vi "PH_Sixpack.Action Reset.vi"(0 "i ref in":refnum<vi>, 5 "error in":errorcluster) -> (14 "i ref out":refnum<vi>, 19 "error out":errorcluster)   [LabVIEW 2014, in "PH_Sixpack.lvlib"]
doc: "This VI resets the 6P."
uses:
  PH_Sixpack.lvlib
  PH_Sixpack.Status.ctl
  instr.lib/SixPack/Sixpack - Driver.lvlib
  PH_Stepmotor_BaseClass/PH_Stepmotor_BaseClass.lvlib
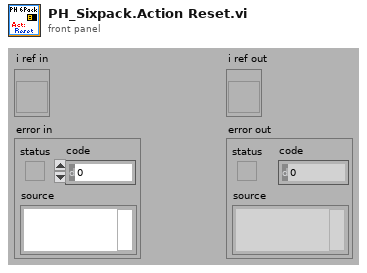
[diagram p1: front panel]
types:
  T1 = typedef "PH_Sixpack.lvlib/PH_Sixpack.Status.ctl" = enum32{"None", "Init", "Configure", "configured", "Close", "closed"}
  T2 = typedef "PH_Stepmotor_BaseClass.lvlib/PH_Stepmotor_BaseClass.i attribute.ctl" = cluster{"Device Error":errorcluster, "Axes PSDB Thread":cluster{"Ref":refnum<vi>, "Q-Ref":refnum<queue>, "Data Status":T3}, "Axes":T4[], "Axes PSDB Infos":cluster{"GUI Name":string, "PSDB Instance ID":i32, "PSDB Status Service ID":i32, "Axis":i32, "Class":string}[], "GUI Refs":T9}
  T3 = typedef "PH_PSDBWriter.lvlib/PH_PSDBWriter.Data Status.ctl" = i16
  T4 = typedef "PH_Stepmotor_BaseClass.lvlib/PH_Stepmotor_BaseClass.Axis Attributes.ctl" = cluster{"Settings":T5, "Endswitch?":bool, "DIM Service IDs":T7, "Activity":T8, "Configured?":bool, "Position":cluster{"Current":i32, "Target":i32}, "Position to set":cluster{"New?":bool, "Wanted":i32}, "Stop?":bool, "Reset?":bool, "Move?":bool, "Nothing connected?":bool}
  T5 = typedef "PH_Stepmotor_BaseClass.lvlib/PH_Stepmotor_BaseClass.Axis Settings.ctl" = cluster{"Sign change":bool, "Width":dbl, "Calibration":dbl, "Unit":string, "Motor Type":T6, "Unit Width":string, "Unit CF":string}
  T6 = typedef "PH_Stepmotor_BaseClass.lvlib/PH_Stepmotor_BaseClass.Motor Type.ctl" = enum16{"Unspecific", "OWIS 49.120.2633", "OWIS 49.060.1033", "OWIS 43.040.2558", "Diamond Motion 2200 series", "OWIS 49.120.266B.MV6", "Calorimeter", "Linear Stage 1", "MICOS VT-80", "MICOS VT-80 S", "Standa Rotstage nt0.95A", "PUF RA 320.200", "PUF RA 800.200", "PUF RA 800.400", "PUF RA 400.50", "1324.nn.800.50", "1324.n9c.800.50", "1324.nn.320.200", "1324.nn.400.200", "1324.nn.800.200", "1324.nn.400.50", "1324.8c9c.800.50", "1324.8c9c.400.200"}
  T7 = typedef "PH_Stepmotor_BaseClass.lvlib/PH_Stepmotor_BaseClass.Axis DIM Service IDs.ctl" = cluster{"Settings":i32, "Information":i32}
  T8 = typedef "PH_Stepmotor_BaseClass.lvlib/PH_Stepmotor_BaseClass.Axis Activity.ctl" = enum16{"No Information", "stopped", "running", "Failure", "Alarm", "stopped at backward ES", "stopped at foreward ES"}
  T9 = typedef "PH_Stepmotor_BaseClass.lvlib/PH_Stepmotor_BaseClass.GUI Refs.ctl" = cluster{"Axes Configuration":refnum<vi>, "Device Error":refnum<vi>, "Axes PSDB Infos":refnum<vi>}
  T10 = typedef "PH_Sixpack.lvlib/PH_Sixpack.i attribute.ctl" = cluster{"Information":cluster{"SixPack ID(0)":u16, "BaudRate(19200)":u16, "COM Port":enum32{"COM1", "COM2", "COM3", "COM4", "COM5", "COM6", "COM7", "COM8", "COM9"}, "HANDLE":i32}, "Serial Number":dbl, "Firmwareversion":dbl, "Axes":T11[], "Status":T1, "Axis to do a RefSearch":i32, "GUI Refs":cluster{"Information":refnum<vi>, "Serial Number":refnum<vi>, "Firmwareversion":refnum<vi>, "Status":refnum<vi>, "Axis to do a RefSearch":refnum<vi>, "Axes Configuration (Sixpack)":refnum<vi>, "Inputs":refnum<vi>, "PeriodicInterval [ms]":refnum<vi>}, "Constructor finished":bool, "Ignore Error":bool}
  T11 = typedef "PH_Sixpack.lvlib/PH_Sixpack.Axis Cluster.ctl" = cluster{"Config":T12, "To set?":cluster{"VmaxAmax":bool, "I max":bool, "VStartVminDivi":bool, "Ref Search Parameter":bool, "Stopswitch Limits":bool, "Axis Parameter":bool, "I Control":bool}}
  T12 = typedef "PH_Sixpack.lvlib/PH_Sixpack.Axis Configuration.ctl" = cluster{"VmaxAmax":T13, "I max (50%)":T14, "VStartVminDivi":T15, "Ref Search Parameter":T16, "Stopswitch Limits":T17, "Axis Parameter":T18, "I Control":T21}
  T13 = typedef "Sixpack - Driver.lvlib/VmaxAmax.ctl" = cluster{"VMax(511)":u16, "AMax(128)":u16}
  T14 = typedef "Sixpack - Driver.lvlib/PeakCurrent.ctl" = dbl
  T15 = typedef "Sixpack - Driver.lvlib/VStartVmin.ctl" = cluster{"VStart(5)":u16, "Vmin(4)":u16, "Div i (2)":enum8{"0", "1", "2", "3"}}
  T16 = typedef "Sixpack - Driver.lvlib/Ref Search Parameter.ctl" = cluster{"VRefMax(100)":u16, "DebouncingTime (22ms)":u8}
  T17 = typedef "Sixpack - Driver.lvlib/Stopswitch Limits.ctl" = cluster{"MinLeft(0)":u16, "MaxRight(1023)":u16}
  T18 = typedef "Sixpack - Driver.lvlib/Motor Parameter.ctl" = cluster{"Poslimit (6400)":u32, "P5 Bits":T19, "P6 Bits":T20}
  T19 = typedef "Sixpack - Driver.lvlib/MotorParameter_P5.ctl" = cluster{"MT_PI":bool, "MT_ROTARY":bool, "MT_AUTONULLCMD":bool, "MT_TESTNULL":bool, "MT_NULLLEFT":bool, "MT_NULLCENTRE":bool, "MT_STOPNULL":bool, "MT_FILTERSWITCH":bool}
  T20 = typedef "Sixpack - Driver.lvlib/MotorParameter_P6.ctl" = cluster{"MT_OPTIMIZEWAY":bool, "MT_FASTREF":bool, "MT_MECHREF":bool, "MT_DELAYTESTNULL":bool, "MT_STOPSOFT":bool, "MT_STOPNOREF":bool, "MT_NULLPOSITIVE":bool, "MUT_STOPFULSTEPS":bool}
  T21 = typedef "Sixpack - Driver.lvlib/Current Control.ctl" = cluster{"PowerDownDelay (500)":u16, "PowerDown (0%)":T22, "Standing (50%)":T22, "Running (75%)":T22, "Accelerating (100%)":T22}
  T22 = typedef "Sixpack - Driver.lvlib/Current.ctl" = enum8{"100%", "75%", "50%", "38%", "25%", "19%", "13%", "9%", "0%"}
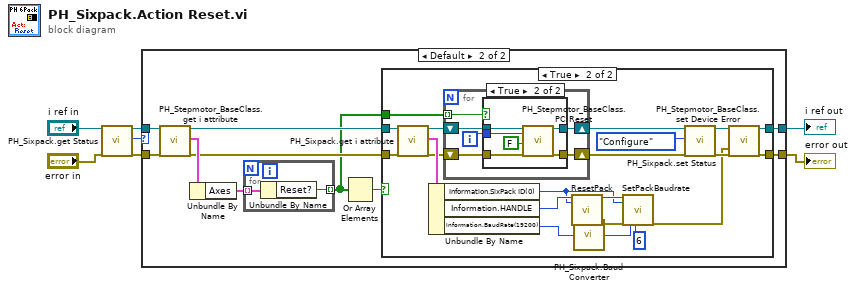
[diagram p0: block diagram]
diagram:
  n1 = call "PH_Sixpack.get Status.vi"("VI in"="i ref in", "error in (no error)"="error in") -> ("VI out"=w4:refnum<vi>, "Status"=w1:T1, "error out"=w2:errorcluster)  [unwired: 14 in, 1 out]
  n2 = case shown="Default" w1 {
    tunnel: [w9 w19] -> w7
    tunnel: [w8 w18] -> w6
    tunnel: w4 -> [w9 w11]
    tunnel: w2 -> [w8 w10]
    frame "None" {
    }
    frame Default {
      n3 = call "PH_Stepmotor_BaseClass.get i attribute.vi"("i ref in"=w11, "error in (no error)"=w10) -> ("i ref out"=w15:refnum<vi>, "i attribute"=w17:T2, "error out"=w14:errorcluster)  [unwired: 15 in]
      n4 = Unbundle By Name(w17) -> ("Axes"=w16:T4[])
      n5 = for {
        tunnel: w16 -> [w58] mode=indexing
        tunnel: [w57] -> w12 mode=indexing
        n6 = Unbundle By Name(w58) -> ("Reset?"=w57:bool)
      }
      n7 = Or Array Elements(Boolean array=w12) -> (logical OR=w13:bool)
      n8 = case shown="True" w13 {
        tunnel: [w21 w25] -> w19
        tunnel: [w20 w23] -> w18
        tunnel: w15 -> [w21 w34]
        tunnel: w14 -> [w20 w33]
        tunnel: w12 -> [_ w30]
        frame False {
        }
        frame True {
          n9 = call "PH_Sixpack.get i attribute.vi"("i ref in"=w34, "error in (no error)"=w33) -> ("i ref out"=w32:refnum<vi>, "i attribute"=w42:T10, "error out"=w31:errorcluster)  [unwired: 15 in]
          n10 = Unbundle By Name(w42) -> ("Information.SixPack ID(0)"=w35:u16, "Information.HANDLE"=w40:i32, "Information.BaudRate(19200)"=w41:u16)
          n11 = for {
            shift-right: [w47] -> w28
            shift-left: w32 -> [w48]
            shift-right: [w45] -> w29
            shift-left: w31 -> [w46]
            tunnel: w30 -> [w43] mode=indexing
            i -> [w44]
            n12 = case shown="True" w43 {
              tunnel: w48 -> [w50 w56]
              tunnel: [w50 w55] -> w47
              tunnel: w46 -> [w49 w54]
              tunnel: [w49 w53] -> w45
              tunnel: w44 -> [_ w52]
              frame False {
              }
              frame True {
                n13 = call "PH_Stepmotor_BaseClass.PC Reset.vi"("i ref in"=w56, "axis"=w52, "Reset?"=FALSE, "error in (no error)"=w54) -> ("i ref out"=w55:refnum<vi>, "error out"=w53:errorcluster)  [unwired: 14 in]
              }
            }
          }
          n14 = call "ResetPack.vi"("handle in"=w40, "UnitAddress(0)"=w35) -> ("handle out"=w37:i32, "error out"=w38:errorcluster)  [unwired: 16 in]
          n15 = call "PH_Sixpack.Baud Converter.vi"("BaudRate(19200)"=w41) -> ("BaudRate (19200)"=w36:enum32{"9600", "19200", "38400", "57600"})
          n16 = call "SetPackBaudrate.vi"("handle in"=w37, "UnitAddress(0)"=w35, "error in"=w38, "BaudRate (19200)"=w36, "Delay(6)"=u16 6 ("Delay")) -> ("error out"=w22:errorcluster)  [unwired: 13 in, 1 out]
          n17 = call "PH_Sixpack.set Status.vi"("VI in"=w28, "Status"=PH_Sixpack.Status."Configure", "error in (no error)"=w29) -> ("VI out"=w26:refnum<vi>, "error out"=w24:errorcluster)  [unwired: 15 in]
          n18 = call "PH_Stepmotor_BaseClass.set Device Error.vi"("i ref in"=w26, "Device Error"=w22, "error in"=w24) -> ("i ref out"=w25:refnum<vi>, "error out"=w23:errorcluster)  [unwired: 15 in]
        }
      }
    }
  }
  "error out" <- w6
  "i ref out" <- w7
